vi "Neocera21 Get H.vi"(8 "error in (no error)":errorcluster, 11 "VISA Resource Name":refnum<visa-resource-name>) -> (0 "error out":errorcluster, 1 "Heater power":dbl, 2 "data string":string, 3 "VISA Resource Name Out":refnum<visa-resource-name>, 4 "Heat %":dbl format="%.2f", 5 "Heater range":i32)   [LabVIEW 2015]
uses:
  GPIB/VISA  Send Receive.vi
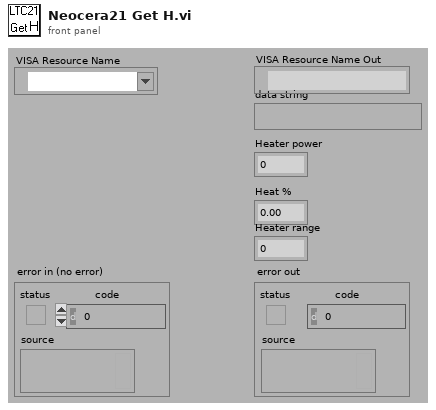
[diagram p1: front panel]
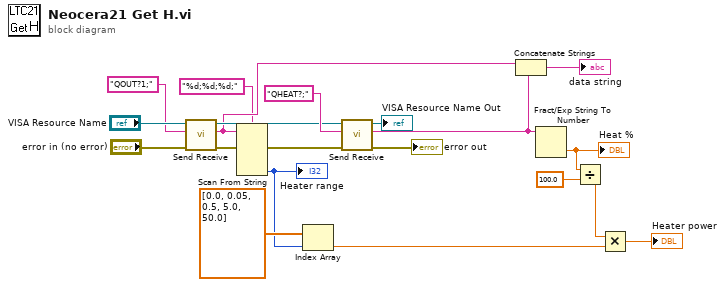
[diagram p0: block diagram]
diagram:
  n1 = call-poly "Send Receive.vi"("error in (no error)"="error in (no error)", "data string in"="QOUT?1;" ("data string"), "VISA Resource Name"="VISA Resource Name") -> ("error out"=w2:errorcluster, "data string out"=w11:string, "VISA Resource Name Out"=w14:refnum<visa-resource-name>)  [unwired: 6 in]
  n2 = Scan From String(format string="%d;%d;%d;", input string=w11, error in=w2) -> (error out=w1:errorcluster, output 3=w8:i32)  [unwired: 6 in, 2 out]
  "Heater range" <- w8
  n3 = Index Array(array=dbl[] [0.0, 0.05, 0.5, 5.0, 50.0], index=w8) -> (element=w7:dbl)
  n4 = call-poly "Send Receive.vi"("error in (no error)"=w1, "data string in"="QHEAT?;" ("data string"), "VISA Resource Name"=w14) -> ("error out"=→"error out":errorcluster, "data string out"=w19:string, "VISA Resource Name Out"=→"VISA Resource Name Out":refnum<visa-resource-name>)  [unwired: 6 in]
  n5 = Concatenate Strings(w11, w19) -> (→"data string":string)
  n6 = Fract/Exp String To Number(string=w19) -> (number=w5:dbl)  [unwired: 3 in, 1 out]
  "Heat %" <- w5
  n7 = Divide(x=w5, y=100.0) -> (x/y=w3:dbl)
  n8 = Multiply(x=w3, y=w7) -> (x*y=→"Heater power":dbl)
